vi "Open Web Service.vi"(8 "error in (no error)":errorcluster, 10 "Proxy Server Settings":T1, 11 "Web Service Authentication":T2) -> (0 "error out":errorcluster, 3 "ContactAndRegisterWithNmaSapService refnum":refnum<k24>)   [LabVIEW 2023, in "ContactAndRegisterWithNmaSapService.lvlib"]
uses:
  <userlib>/WebService/_ContactAndRegisterWithNmaSapService/ContactAndRegisterWithNmaSapService.dll
  <userlib>/WebService/_ContactAndRegisterWithNmaSapService/ContactAndRegisterWithNmaSapService.lvlib
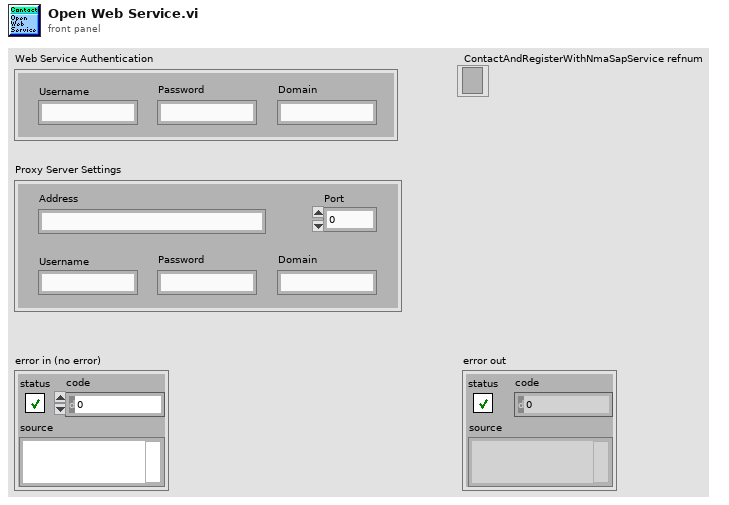
[diagram p1: front panel]
types:
  T1 = cluster{"Address":string, "Port":u32, "Username":string, "Password":string, "Domain":string}
  T2 = cluster{"Username":string, "Password":string, "Domain":string}
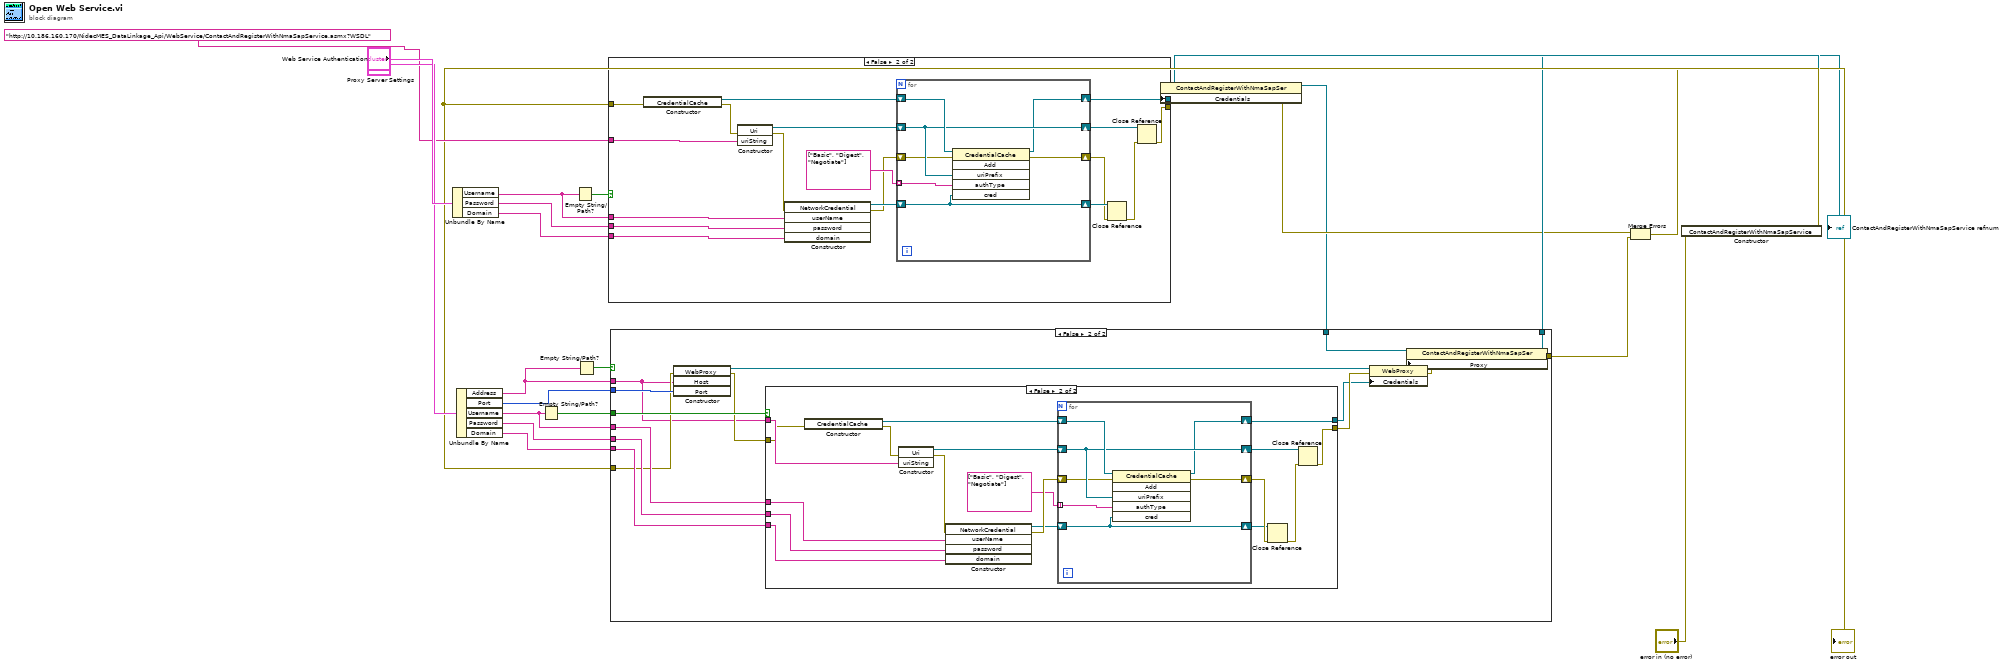
[diagram p0: block diagram]
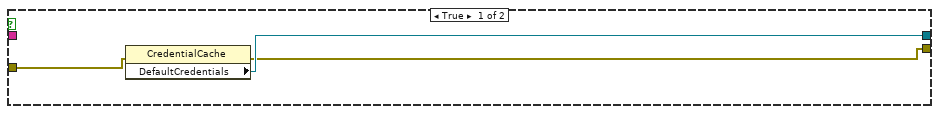
[diagram p3: hidden frame]
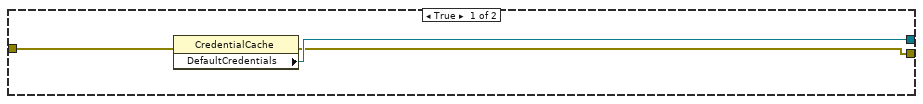
[diagram p4: hidden frame]
diagram:
  n1 = Unbundle By Name("Web Service Authentication") -> ("Username"=w2:string, "Password"=w3:string, "Domain"=w4:string)
  n2 = Unbundle By Name("Proxy Server Settings") -> ("Address"=w7:string, "Port"=w8:u32, "Username"=w12:string, "Password"=w10:string, "Domain"=w11:string)
  n3 = Empty String/Path?(string/path=w12) -> (empty?=w9:bool)
  n4 = Empty String/Path?(string/path=w2) -> (empty?=w1:bool)
  n5 = Empty String/Path?(string/path=w7) -> (empty?=w6:bool)
  n6 = constructor class="ContactAndRegisterWithNmaSapSer"(error in="error in (no error)") -> (reference out=w17:refnum<k24>, error out=w19:errorcluster)  [unwired: 2 in, 1 out]
  n7 = case shown="False" w1 {
    tunnel: w19 -> [w26 w44]
    tunnel: "http://10.186.160.170/NidecMES_DataLinkage_Api/WebService/ContactAndRegisterWithNmaSapService.asmx?WSDL" ("WSDL URL") -> [_ w42]
    tunnel: w2 -> [_ w41]
    tunnel: w3 -> [_ w40]
    tunnel: w4 -> [_ w39]
    tunnel: [w24 w28] -> _
    tunnel: [w25 w27] -> w5
    frame True {
      n8 = property class="CredentialCache"(error in=w26) -> (error out=w24:errorcluster, "DefaultCredentials"=w25:refnum<k24>)  [unwired: 1 in, 1 out]
    }
    frame False {
      n9 = constructor class="CredentialCache"(error in=w44) -> (reference out=w36:refnum<k24>, error out=w43:errorcluster)  [unwired: 2 in, 1 out]
      n10 = constructor class="Uri"(error in=w43, "uriString"=w42) -> (reference out=w35:refnum<k24>, error out=w38:errorcluster)  [unwired: 2 in, 2 out]
      n11 = constructor class="NetworkCredential"(error in=w38, "userName"=w41, "password"=w40, "domain"=w39) -> (reference out=w34:refnum<k24>, error out=w33:errorcluster)  [unwired: 2 in, 4 out]
      n12 = for {
        tunnel: string[] ["Basic", "Digest", "Negotiate"] -> [w46] mode=indexing
        shift-right: [w47] -> w29
        shift-left: w33 -> [w48]
        shift-right: [w50] -> w31
        shift-left: w35 -> [w50]
        shift-right: [w49] -> w27
        shift-left: w36 -> [w51]
        shift-right: [w45] -> w32
        shift-left: w34 -> [w45]
        n13 = invoke class="CredentialCache" method="Add"(reference=w51, error in=w48, "uriPrefix"=w50, "authType"=w46, "cred"=w45) -> (reference out=w49:refnum<k24>, error out=w47:errorcluster)  [unwired: 1 in, 4 out]
      }
      n14 = Close Reference(reference=w32, error in (no error)=w29) -> (error out=w30:errorcluster)
      n15 = Close Reference(reference=w31, error in (no error)=w30) -> (error out=w28:errorcluster)
    }
  }
  n16 = property class="ContactAndRegisterWithNmaSapSer"(reference=w17, "Credentials"=w5) -> (reference out=w13:refnum<k24>, error out=w14:errorcluster)  [unwired: 1 in]
  n17 = case shown="False" w6 {
    tunnel: w7 -> [_ w62]
    tunnel: w8 -> [_ w69]
    tunnel: w9 -> [_ w68]
    tunnel: w10 -> [_ w66]
    tunnel: w11 -> [_ w65]
    tunnel: w12 -> [_ w67]
    tunnel: w19 -> [w52 w64]
    tunnel: w13 -> [w53 w58]
    tunnel: [w53 w56] -> w16
    tunnel: [w52 w55] -> w15
    frame True {
    }
    frame False {
      n18 = constructor class="WebProxy"(error in=w64, "Host"=w62, "Port"=w69) -> (reference out=w59:refnum<k24>, error out=w63:errorcluster)  [unwired: 2 in, 3 out]
      n19 = case shown="False" w68 {
        tunnel: w67 -> [_ w77]
        tunnel: w66 -> [_ w76]
        tunnel: w65 -> [_ w75]
        tunnel: w63 -> [w72 w78]
        tunnel: w62 -> [_ w79]
        tunnel: [w70 w74] -> w61
        tunnel: [w71 w73] -> w60
        frame True {
          n20 = property class="CredentialCache"(error in=w72) -> (error out=w70:errorcluster, "DefaultCredentials"=w71:refnum<k24>)  [unwired: 1 in, 1 out]
        }
        frame False {
          n21 = constructor class="CredentialCache"(error in=w78) -> (reference out=w83:refnum<k24>, error out=w80:errorcluster)  [unwired: 2 in, 1 out]
          n22 = constructor class="Uri"(error in=w80, "uriString"=w79) -> (reference out=w84:refnum<k24>, error out=w81:errorcluster)  [unwired: 2 in, 2 out]
          n23 = constructor class="NetworkCredential"(error in=w81, "userName"=w77, "password"=w76, "domain"=w75) -> (reference out=w85:refnum<k24>, error out=w86:errorcluster)  [unwired: 2 in, 4 out]
          n24 = for {
            tunnel: string[] ["Basic", "Digest", "Negotiate"] -> [w92] mode=indexing
            shift-right: [w93] -> w90
            shift-left: w86 -> [w94]
            shift-right: [w96] -> w88
            shift-left: w84 -> [w96]
            shift-right: [w95] -> w73
            shift-left: w83 -> [w97]
            shift-right: [w91] -> w87
            shift-left: w85 -> [w91]
            n25 = invoke class="CredentialCache" method="Add"(reference=w97, error in=w94, "uriPrefix"=w96, "authType"=w92, "cred"=w91) -> (reference out=w95:refnum<k24>, error out=w93:errorcluster)  [unwired: 1 in, 4 out]
          }
          n26 = Close Reference(reference=w87, error in (no error)=w90) -> (error out=w89:errorcluster)
          n27 = Close Reference(reference=w88, error in (no error)=w89) -> (error out=w74:errorcluster)
        }
      }
      n28 = property class="WebProxy"(reference=w59, error in=w61, "Credentials"=w60) -> (reference out=w54:refnum<k24>, error out=w57:errorcluster)
      n29 = property class="ContactAndRegisterWithNmaSapSer"(reference=w58, error in=w57, "Proxy"=w54) -> (reference out=w56:refnum<k24>, error out=w55:errorcluster)
    }
  }
  "ContactAndRegisterWithNmaSapService refnum" <- w16
  n30 = Merge Errors(w14, w15) -> (→"error out":errorcluster)
